vi "Release Aquirer.vi"(8 "error in (no error)":errorcluster, 10 "Aquirer Index":i32, 11 "Instrument Handler in":refnum<class "Instrument Handler.lvclass">) -> (0 "error out":errorcluster, 3 "Instrument Handler out":refnum<class "Instrument Handler.lvclass">)   [LabVIEW 2020, in "Instrument Handler.lvlib" / "Instrument Handler.lvclass"]
doc: "Release an Aquirer by index."
uses:
  Instrument Handler.lvclass
  Instrument Handler.lvclass/Instrument Handler.ctl
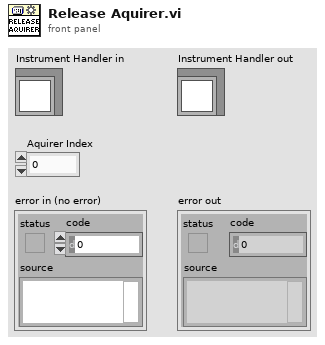
[diagram p1: front panel]
types:
  T1 = typedef "Instrument Handler.lvlib/Ctl_AquirerAvailabilityStatus.ctl" = cluster{"Available?":bool, "Aquirer":T2}
  T2 = typedef "Instrument Handler.lvlib/Ctl_AquirerRefnum.ctl" = refnum<vi>
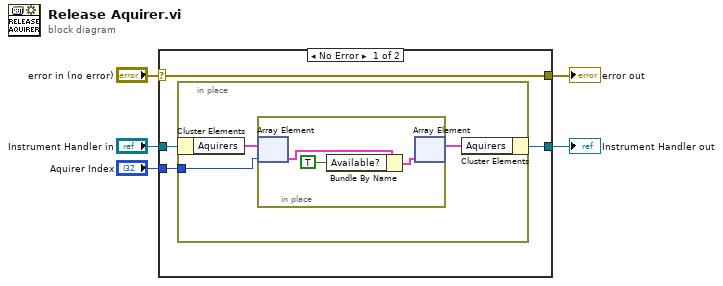
[diagram p0: block diagram]
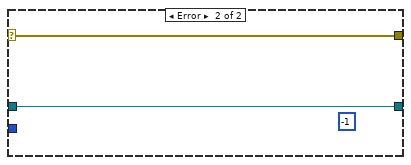
[diagram p2: hidden frame]
diagram:
  n1 = case shown="No Error" "error in (no error)" {
    selector: "error in (no error)" -> [w6 w17]
    tunnel: [w6 w17] -> w4
    tunnel: [w8 w16] -> w2
    tunnel: "Instrument Handler in" -> [w9 w16]
    tunnel: "Aquirer Index" -> [w7 _]
    frame No Error {
      n2 = in-place {
        in-place-border: w7 -> [w10]
        n3 = in-place-cluster #1(w9) -> ("Aquirers"=w12:T1[])
        n4 = in-place {
          n5 = in-place-array #2(w12, w10) -> (w15:T1)
          n6 = Bundle By Name(cluster=w15, "Available?"=TRUE) -> (w13:T1)
          n7 = in-place-array #2(w13) -> (w11:T1[])  [unwired: 1 out]
        }
        n8 = in-place-cluster #1("Aquirers"=w11) -> (w8:refnum<class "Instrument Handler.lvclass">)
      }
    }
    frame Error {
      (unwired) -1
    }
  }
  "error out" <- w4
  "Instrument Handler out" <- w2
